vi "平行样测试数据写入.vi"(8 "error in (no error)":errorcluster, 11 "data":T1={"时间标识"=timestamp(0 s since 1904-01-01), "参数"="", "数据类型"="N", "第一次水样浓度值"=0.0, "第二次水样测试时间"=timestamp(0 s since 1904-01-01), "第二次水样浓度值"=0.0}) -> (0 "error out":errorcluster)   [LabVIEW 2016, in "质控单元.lvlib"]
uses:
  <vilib>/addons/database/Auxilliary.llb/DB Tools Column Info.ctl
  <vilib>/addons/database/Auxilliary.llb/DB Tools DataTypes.ctl
  <vilib>/addons/database/NI_Database_API.lvlib
panel:
  out "输出簇":T1
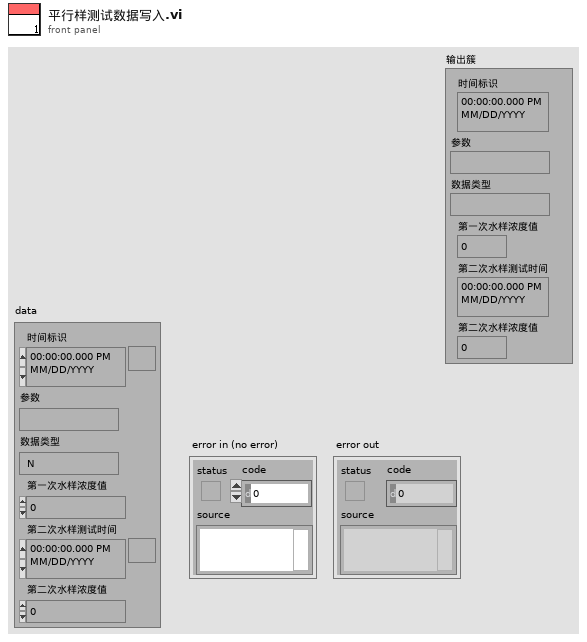
[diagram p1: front panel]
types:
  T1 = cluster{"时间标识":timestamp, "参数":string, "数据类型":string, "第一次水样浓度值":sgl, "第二次水样测试时间":timestamp, "第二次水样浓度值":sgl}
  T2 = typedef "NI_Database_API.lvlib/DB Tools Column Info.ctl" = cluster{"column name":string, "data type":T3, "size":i32, "allow null?":bool}
  T3 = typedef "NI_Database_API.lvlib/DB Tools DataTypes.ctl" = enum16{"String", "Long (I32)", "Single (SGL)", "Double (DBL)", "Date/Time", "Binary"}
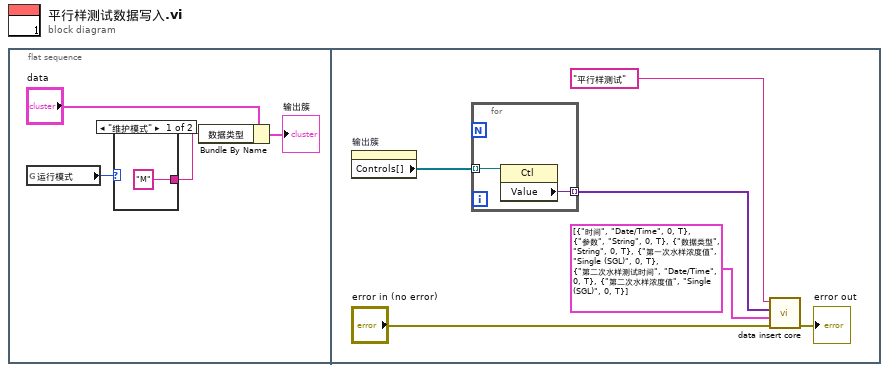
[diagram p0: block diagram]
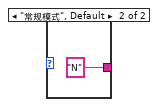
[diagram p2: hidden frame]
diagram:
  n1 = flat-sequence {
    frame #0 {
      n2 = global read "系统交互.vi" "运行模式"() -> (w3:enum16{"维护模式", "常规模式", "应急模式", "质控模式"})
      n3 = case shown="\"维护模式\"" w3 {
        tunnel: ["M" "N"] -> w4
        frame "维护模式" {
        }
        frame "常规模式", Default {
        }
      }
      n4 = Bundle By Name(cluster="data", "数据类型"=w4) -> (→"输出簇":T1)
    }
    frame #1 {
      n5 = property on="输出簇" class="Clust (严格)"() -> ("Controls[]"=w9:refnum<vi>[])  [unwired: 2 in, 2 out]
      n6 = for {
        tunnel: w9 -> [w14] mode=indexing
        tunnel: [w13] -> w8 mode=indexing
        n7 = property class="Ctl"(reference=w14) -> ("Value"=w13:variant)  [unwired: 1 in, 2 out]
      }
      n8 = call "data insert core.vi"("error in (no error)"="error in (no error)", "column information"=T2[] [{"column name"="时间", "data type"=enum."Date/Time", "size"=0, "allow null?"=TRUE}, {"column name"="参数", "data type"=enum."String", "size"=0, "allow null?"=TRUE}, {"column name"="数据类型", "data type"=enum."String", "size"=0, "allow null?"=TRUE}, {"column name"="第一次水样浓度值", "data type"=enum."Single (SGL)", "size"=0, "allow null?"=TRUE}, {"column name"="第二次水样测试时间", "data type"=enum."Date/Time", "size"=0, "allow null?"=TRUE}, {"column name"="第二次水样浓度值", "data type"=enum."Single (SGL)", "size"=0, "allow null?"=TRUE}], "data"=w8, "table"="平行样测试") -> ("error out"=→"error out":errorcluster)  [unwired: 7 in]
    }
  }
